vi "TCP-IP Link.Send.vi"(8 "error in":errorcluster, 10 "Data":string, 11 "Link Q Name":string="TCP-IP_Link") -> (0 "error out":errorcluster)   [LabVIEW 2024, in "EQMF.lvlib" / "TCP-IP.lvlib"]
uses:
  TCP-IP.lvlib
  Queues/Queue Utils.lvlib
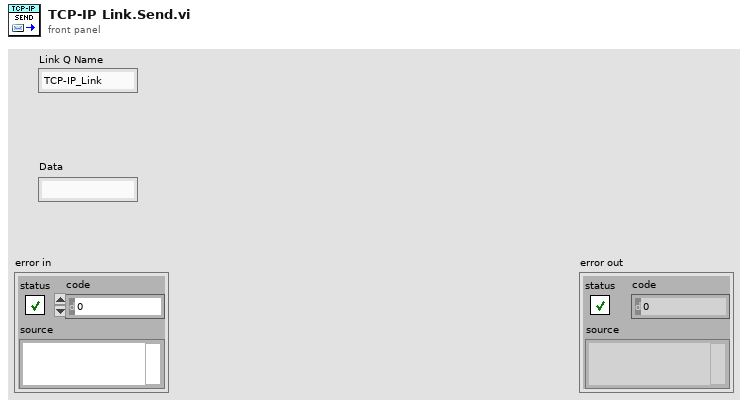
[diagram p1: front panel]
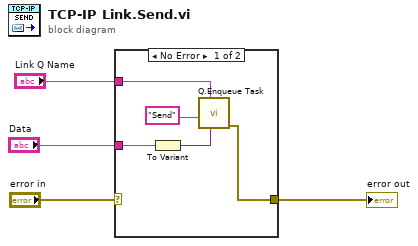
[diagram p0: block diagram]
diagram:
  n1 = case shown="No Error" "error in" {
    selector: "error in" -> [_ w10]
    tunnel: "Link Q Name" -> [w7 _]
    tunnel: "Data" -> [w6 _]
    tunnel: [w5 w10] -> w1
    frame No Error {
      n2 = To Variant(anything=w6) -> (Variant=w8:variant)
      n3 = call "Q.Enqueue Task.vi"("Data1"=w8, "Q Name"=w7, "Task Name"="Send") -> ("error out"=w5:errorcluster)  [unwired: 7 in, 1 out]
    }
    frame Error {
    }
  }
  "error out" <- w1
